vi "Form Message for Level and Limit Errors.vi"(2 "Pin Names[]":string[](array[string]), 7 "Limit Errors[]":errorcluster[](array[cluster]), 9 "Level Error[]":errorcluster[](array[cluster]), 11 "error in":errorcluster) -> (6 "Error Pins":string, 15 "error out":errorcluster)   [LabVIEW 2024, in "devicePowerSequencerCoreLogic.lvlib"]
uses:
  devicePowerSequencerCoreLogic.lvlib
  <vilib>/Utility/error.llb/Trim Whitespace One-Sided.vi
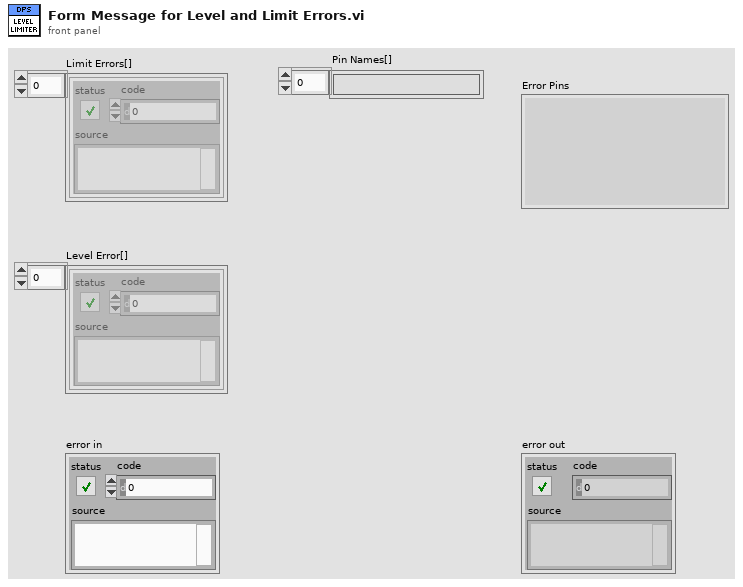
[diagram p1: front panel]
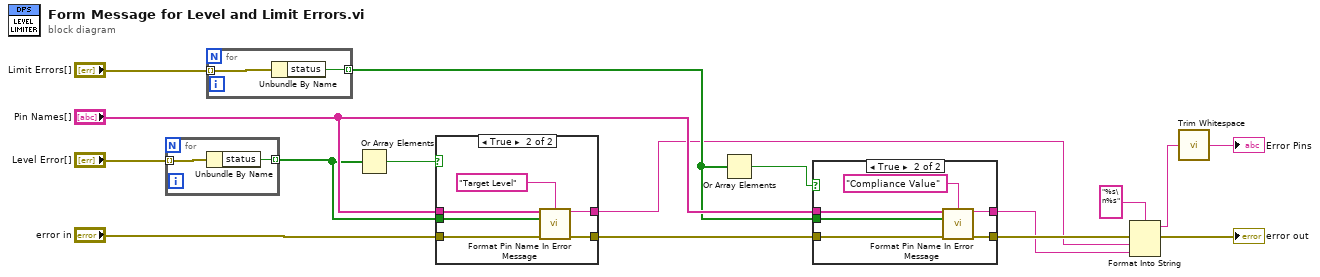
[diagram p0: block diagram]
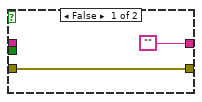
[diagram p2: hidden frame]
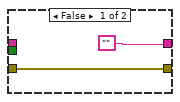
[diagram p3: hidden frame]
diagram:
  n1 = for {
    tunnel: "Level Error[]" -> [w18] mode=indexing
    tunnel: [w17] -> w10 mode=indexing
    n2 = Unbundle By Name(w18) -> ("status"=w17:bool)
  }
  n3 = for {
    tunnel: "Limit Errors[]" -> [w20] mode=indexing
    tunnel: [w19] -> w8 mode=indexing
    n4 = Unbundle By Name(w20) -> ("status"=w19:bool)
  }
  n5 = Or Array Elements(Boolean array=w10) -> (logical OR=w9:bool)
  n6 = case shown="True" w9 {
    tunnel: "Pin Names[]" -> [_ w27]
    tunnel: [w22 w26] -> w13
    tunnel: "error in" -> [w22 w25]
    tunnel: ["" w24] -> w4
    tunnel: w10 -> [_ w23]
    frame False {
    }
    frame True {
      n7 = call "Format Pin Name In Error Message.vi"("Pin Name"=w27, "Parameter Name"="Target Level", "Error[]"=w23, "error in"=w25) -> ("Error Message"=w24:string, "error out"=w26:errorcluster)  [unwired: 10 in]
    }
  }
  n8 = Or Array Elements(Boolean array=w8) -> (logical OR=w7:bool)
  n9 = case shown="True" w7 {
    tunnel: "Pin Names[]" -> [_ w36]
    tunnel: w13 -> [w30 w34]
    tunnel: [w30 w33] -> w6
    tunnel: ["" w32] -> w3
    tunnel: w8 -> [_ w31]
    frame False {
    }
    frame True {
      n10 = call "Format Pin Name In Error Message.vi"("Pin Name"=w36, "Parameter Name"="Compliance Value", "Error[]"=w31, "error in"=w34) -> ("Error Message"=w32:string, "error out"=w33:errorcluster)  [unwired: 10 in]
    }
  }
  n11 = Format Into String(format string="%s\n%s", error in=w6, w4, w3) -> (resulting string=w2:string, error out=→"error out":errorcluster)  [unwired: 1 in]
  n12 = call <vilib>:"Trim Whitespace.vi"("string"=w2) -> ("trimmed string"=→"Error Pins":string)  [unwired: 1 in]
